vi "Rd Wr Script Defaults.vi"(8 "error in (no error)":errorcluster, 10 "Write? (F:Read)":bool, 11 "Script Settings":T1) -> (0 "error out":errorcluster, 3 "Script Settings":T1)   [LabVIEW 2024]
uses:
  CC cluster Script Panel Defaults.ctl
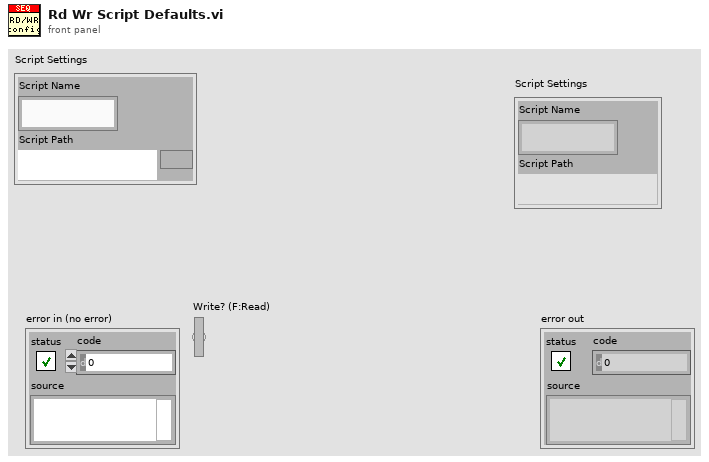
[diagram p1: front panel]
types:
  T1 = typedef "CC cluster Script Panel Defaults.ctl" = cluster{"Script Name":string, "Script Path":path}
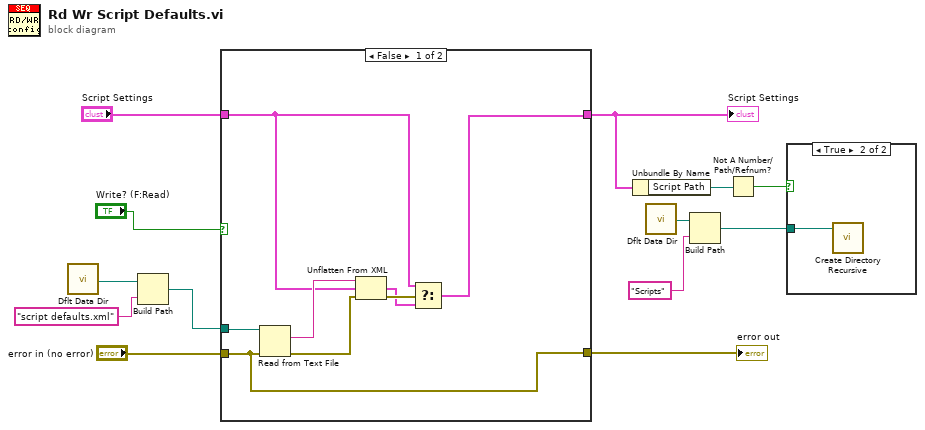
[diagram p0: block diagram]
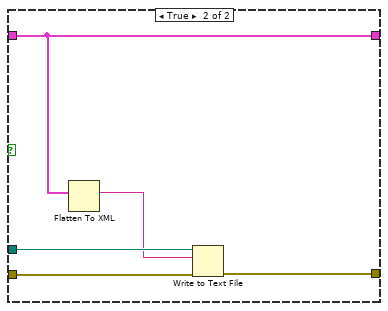
[diagram p3: hidden frame]
diagram:
  n1 = call <vilib>:"Dflt Data Dir.vi"() -> ("App:Default Data Directory"=w10:path)
  n2 = Build Path(base path=w10, name or relative path="script defaults.xml") -> (appended path=w9:path)
  n3 = case shown="False" "Write? (F:Read)" {
    tunnel: "error in (no error)" -> [w15 w26]
    tunnel: "Script Settings" -> [w17 w22]
    tunnel: w9 -> [w21 w25]
    tunnel: [w15 w23] -> w8
    tunnel: [w16 w22] -> w5
    frame False {
      n4 = Read from Text File(file (use dialog)=w21, error in=w15) -> (text=w20:string, error out=w19:errorcluster)  [unwired: 2 in, 2 out]
      n5 = Unflatten From XML(xml string=w20, type=w17, error in (no error)=w19) -> (value=w14:T1, error out=w18:errorcluster)
      n6 = Select(t=w17, s=w18, f=w14) -> (s? t:f=w16:T1)
    }
    frame True {
      n7 = Flatten To XML(6:w22) -> (2:w24:string)
      n8 = Write to Text File(file (use dialog)=w25, text=w24, error in=w26) -> (error out=w23:errorcluster)  [unwired: 1 in, 2 out]
    }
  }
  "error out" <- w8
  "Script Settings" <- w5
  n9 = Unbundle By Name(w5) -> ("Script Path"=w6:path)
  n10 = call <vilib>:"Dflt Data Dir.vi"() -> ("App:Default Data Directory"=w3:path)
  n11 = Build Path(base path=w3, name or relative path="Scripts") -> (appended path=w1:path)
  n12 = Not A Number/Path/Refnum?(number/path/refnum=w6) -> (NaN/Path/Refnum?=w4:bool)
  n13 = case shown="True" w4 {
    tunnel: w1 -> [_ w27]
    frame False {
    }
    frame True {
      n14 = call <vilib>:"Create Directory Recursive.vi"("directory"=w27) -> ()  [unwired: 4 in, 3 out]
    }
  }
